vi "writeToXML.vi"(8 "error in (no error)":errorcluster, 10 "Class Label":string, 11 "CurrentTimes in":refnum<class "CurrentTimes.lvclass">) -> (0 "error out":errorcluster, 2 "XML out":string, 3 "CurrentTimes out":refnum<class "CurrentTimes.lvclass">)   [LabVIEW 2014, in "TCSDataDefinitions.lvlib" / "TCSPublicStatus.lvlib" / "CurrentTimes.lvlib" / "CurrentTimes.lvclass"]
uses:
  CurrentTimes.lvclass
  CurrentTimes.lvclass/CurrentTimes.ctl
  ClockTimes/ClockTimes.lvclass
  <userlib>/Common/XML/XMLGenerator/XMLGenerator.lvclass
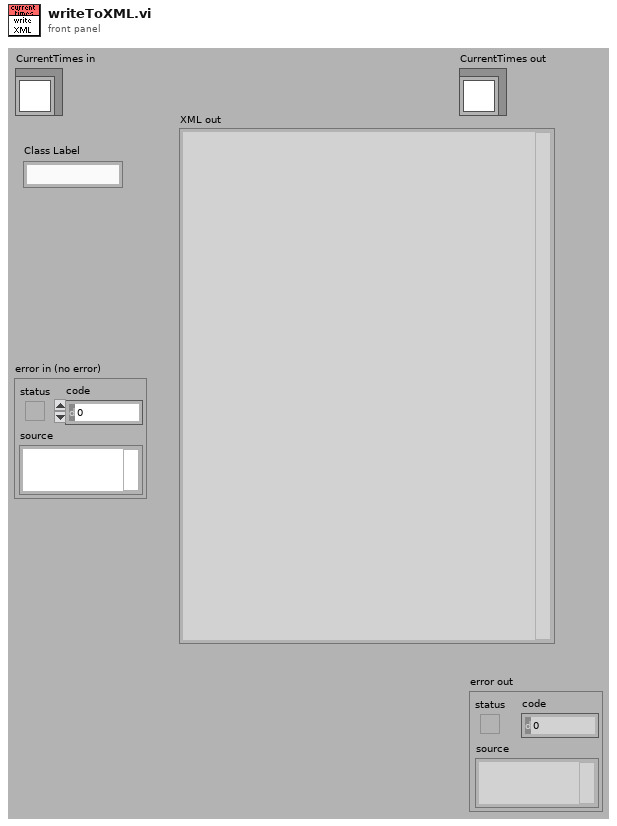
[diagram p1: front panel]
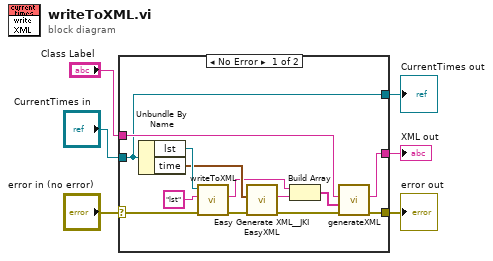
[diagram p0: block diagram]
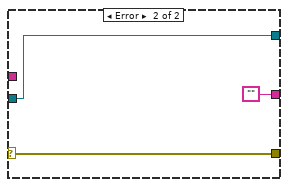
[diagram p2: hidden frame]
diagram:
  n1 = case shown="No Error" "error in (no error)" {
    selector: "error in (no error)" -> [w8 w22]
    tunnel: [w16 w22] -> w5
    tunnel: [w15 w21] -> w3
    tunnel: "CurrentTimes in" -> [w15 w21]
    tunnel: [w18 ""] -> w2
    tunnel: "Class Label" -> [w19 _]
    frame No Error {
      n2 = Unbundle By Name(w15) -> ("lst"=w13:refnum<class "ClockTimes.lvclass">, "time"=w12:timestamp)
      n3 = call-dynamic "writeToXML.vi"("error in (no error)"=w8, "Class Label"="lst", "ClockTimes in"=w13) -> ("error out"=w14:errorcluster, "XML out"=w11:string)  [unwired: 6 in, 1 out]
      n4 = call <vilib>:"Easy Generate XML__JKI EasyXML.vi"("error in (no error)"=w14, "LabVIEW Data"=w12) -> ("error out"=w7:errorcluster, "XML String"=w10:string)  [unwired: 8 in]
      n5 = Build Array(w11, w10) -> (w9:string[])
      n6 = call <userlib>:"generateXML.vi"("error in"=w7, "childrenXML"=w9, "elementName"=w19) -> ("error out"=w16:errorcluster, "XML out"=w18:string)  [unwired: 6 in, 1 out]
    }
    frame Error {
    }
  }
  "error out" <- w5
  "CurrentTimes out" <- w3
  "XML out" <- w2
